vi "MakeExample.vi"(8 "error in (no error)":errorcluster, 9 "TriggerRefractoryPeriod (Frames)":i32, 10 "StimulusObject Parameters":variant, 11 "FullWormRails in":refnum<class "FullWormRails.lvclass">) -> (0 "error out":errorcluster, 3 "FullWormRails out":refnum<class "FullWormRails.lvclass">)   [LabVIEW 2019, in "FullWormRails.lvclass"]
uses:
  FullWormRails.lvclass
  FullWormRailsInputCluster.ctl
  FullWormRails.lvclass/FullWormRails.ctl
  ParametersGlobal.vi
  StimulusObject.lvclass
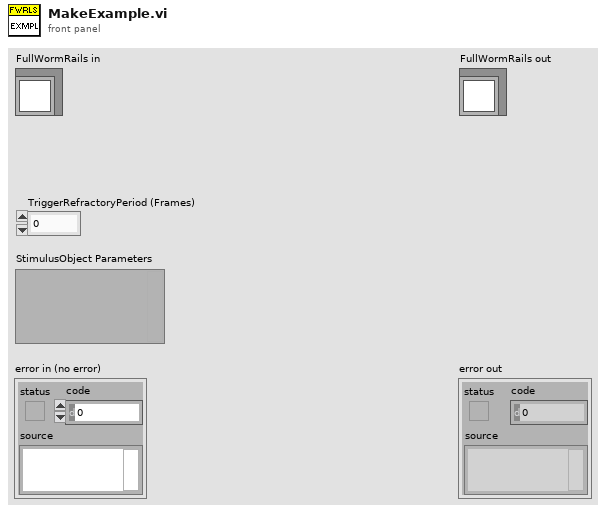
[diagram p1: front panel]
types:
  T1 = typedef "FullWormRails.lvclass/FullWormRailsInputCluster.ctl" = cluster{"Constant Intensity (uW/mm^2, negative is blue)":sgl, "dot radius (mm)":sgl, "Intensities (uW/mm^2, negative is blue)":sgl[], "Durations (s)":sgl[], "Inter trigger interval (s)":dbl}
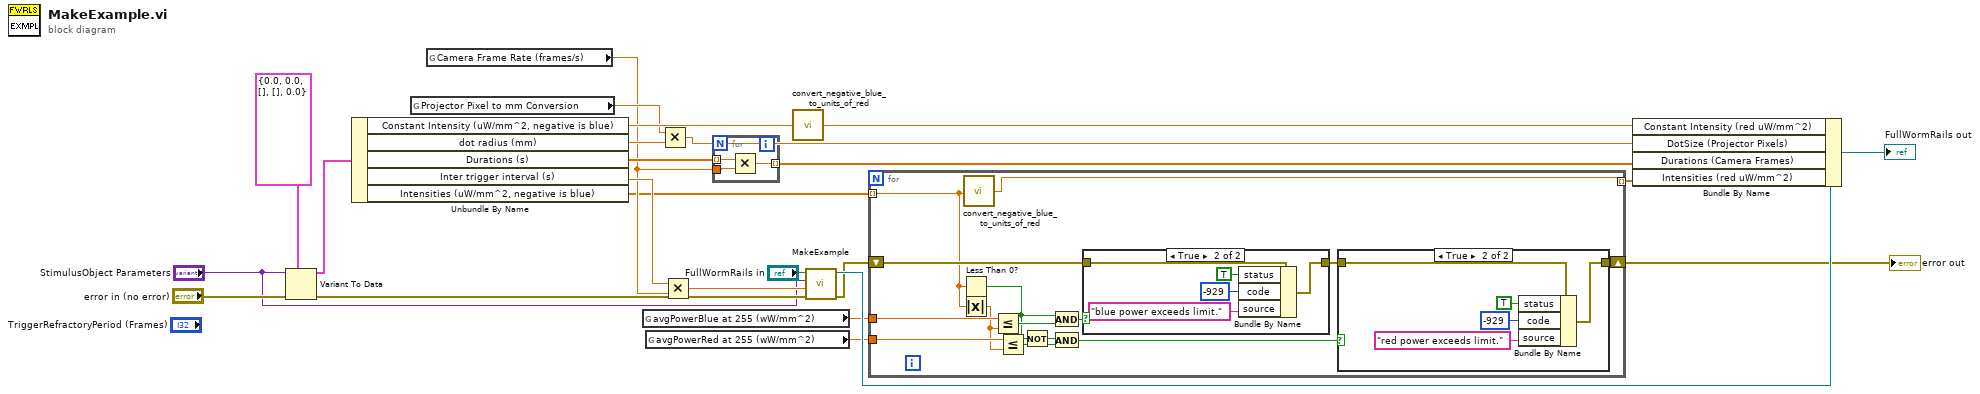
[diagram p0: block diagram]
diagram:
  n1 = Variant To Data(error in="error in (no error)", type=T1 {"Constant Intensity (uW/mm^2, negative is blue)"=0.0, "dot radius (mm)"=0.0, "Intensities (uW/mm^2, negative is blue)"=[], "Durations (s)"=[], "Inter trigger interval (s)"=0.0} ("FullWormRailsInputCluster"), Variant="StimulusObject Parameters") -> (data=w20:T1, error out=w22:errorcluster)
  n2 = Unbundle By Name(w20) -> ("Constant Intensity (uW/mm^2, negative is blue)"=w14:sgl, "dot radius (mm)"=w12:sgl, "Durations (s)"=w9:sgl[], "Inter trigger interval (s)"=w19:dbl, "Intensities (uW/mm^2, negative is blue)"=w6:sgl[])
  n3 = global read "ParametersGlobal.vi" "Projector Pixel to mm Conversion"() -> (w11:sgl)
  n4 = global read "ParametersGlobal.vi" "Camera Frame Rate (frames/s)"() -> (w8:sgl)
  n5 = global read "ParametersGlobal.vi" "avgPowerBlue at 255 (wW/mm^2)"() -> (w4:sgl)
  n6 = global read "ParametersGlobal.vi" "avgPowerRed at 255 (wW/mm^2)"() -> (w3:sgl)
  n7 = Multiply(x=w11, y=w12) -> (x*y=w10:sgl)
  n8 = Multiply(x=w19, y=w8) -> (x*y=w18:dbl)
  n9 = for {
    tunnel: w9 -> [w27] mode=indexing
    tunnel: w8 -> [w26]
    tunnel: [w25] -> w7 mode=indexing
    n10 = Multiply(x=w27, y=w26) -> (x*y=w25:sgl)
  }
  n11 = call "convert_negative_blue_to_units_of_red.vi"("Intensity in units of red (positive) and blue (negative)"=w14) -> ("Intensity in units of red (positive and negative)"=w13:sgl)
  n12 = call-parent "MakeExample.vi"("error in (no error)"=w22, "TriggerRefractoryPeriod (Frames)"=w18, "StimulusObject Parameters"="StimulusObject Parameters", "StimulusObject in"="FullWormRails in") -> ("error out"=w5:errorcluster, "StimulusObject out"=w16:refnum<class "FullWormRails.lvclass">)  [unwired: 6 in]
  n13 = for {
    tunnel: w6 -> [w35] mode=indexing
    shift-right: [w39] -> w1
    shift-left: w5 -> [w40]
    tunnel: w4 -> [w38]
    tunnel: w3 -> [w37]
    tunnel: [w36] -> w2 mode=indexing
    n14 = Less Than 0?(x=w35) -> (x < 0?=w28:bool)
    n15 = Absolute Value(x=w35) -> (abs(x)=w34:sgl)
    n16 = call "convert_negative_blue_to_units_of_red.vi"("Intensity in units of red (positive) and blue (negative)"=w35) -> ("Intensity in units of red (positive and negative)"=w36:sgl)
    n17 = Less Or Equal?(x=w38, y=w34) -> (x <= y?=w33:bool)
    n18 = Less Or Equal?(x=w37, y=w34) -> (x <= y?=w30:bool)
    n19 = Not(x=w28) -> (.not. x?=w29:bool)
    n20 = And(x=w28, y=w33) -> (x .and. y?=w32:bool)
    n21 = And(x=w29, y=w30) -> (x .and. y?=w31:bool)
    n22 = case shown="True" w32 {
      tunnel: w40 -> [w48 w53]
      tunnel: [w48 w52] -> w41
      frame False {
      }
      frame True {
        n23 = Bundle By Name(cluster=w53, "status"=TRUE, "code"=-929, "source"="blue power exceeds limit.") -> (w52:errorcluster)
      }
    }
    n24 = case shown="True" w31 {
      tunnel: w41 -> [w42 w47]
      tunnel: [w42 w46] -> w39
      frame False {
      }
      frame True {
        n25 = Bundle By Name(cluster=w47, "status"=TRUE, "code"=-929, "source"="red power exceeds limit.") -> (w46:errorcluster)
      }
    }
  }
  "error out" <- w1
  n26 = Bundle By Name(cluster=w16, "Constant Intensity (red uW/mm^2)"=w13, "DotSize (Projector Pixels)"=w10, "Durations (Camera Frames)"=w7, "Intensities (red uW/mm^2)"=w2) -> (→"FullWormRails out":refnum<class "FullWormRails.lvclass">)
